vi "CheesyDrive.vi"(6 "Quickturn":bool, 10 "Wheel":dbl(slide) scale=-1.0..1.0, 11 "Throttle":dbl(slide)=-0.0 scale=-1.0..1.0) -> (2 "Right PWM":dbl=0.5949513901284444, 3 "Left PWM":dbl=0.5949513901284444)   [LabVIEW 2017]
doc: "Implements CheesyDrive. CheesyDrive means that the turn joystick controls the radius of turning instead of the rate of turning. Also implements QuickStop and QuickTurn."
panel:
  in  "Slowness":T1={"MaxSpeedSlow"=0.8, "SlowRate"=20.0, "MaxTurnSlow"=0.8, "MaxTurnRateSlow"=20.0}
  in  "PointsTurn":cluster{"X":dbl, "Y":dbl}[](array[cluster])=[{"X"=0.0, "Y"=0.0}, {"X"=0.04, "Y"=0.0}, {"X"=0.041, "Y"=0.01}, {"X"=1.0, "Y"=1.0}, {"X"=1.0, "Y"=1.0}]
  in  "PointsQuickTurn":cluster{"X":dbl, "Y":dbl}[](array[cluster])=[{"X"=0.0, "Y"=0.0}, {"X"=0.04, "Y"=0.0}, {"X"=0.7, "Y"=0.5}, {"X"=1.0, "Y"=1.0}]
  in  "PointsThrottle":cluster{"X":dbl, "Y":dbl}[](array[cluster])=[{"X"=0.0, "Y"=0.0}, {"X"=0.04, "Y"=0.0}, {"X"=0.0251, "Y"=0.15}, {"X"=1.0, "Y"=1.0}]
  in  "CarLikeTurning":bool
  in  "QSMult":dbl=0.1
  in  "WheelNonLinearity":dbl=0.65
  in  "negInertiaScalar":dbl=3.0
  in  "alpha":dbl=0.1
  out "Waveform Chart":dbl(graph)
  in  "Sensitivty":dbl=1.0
  # "Enable to enable"
  # "normal"
  # "(for quickstop decay)"
  # "Switch"
  # "Scale"
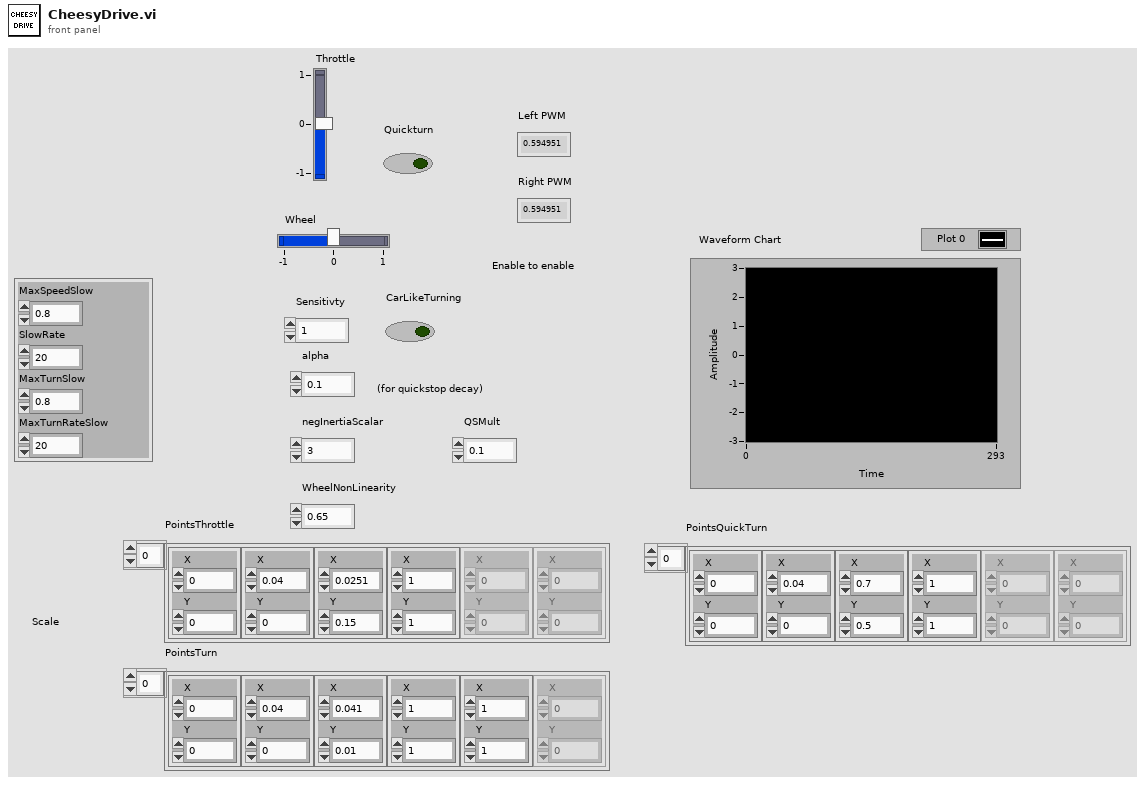
[diagram p1: front panel]
types:
  T1 = cluster{"MaxSpeedSlow":dbl, "SlowRate":dbl, "MaxTurnSlow":dbl, "MaxTurnRateSlow":dbl}
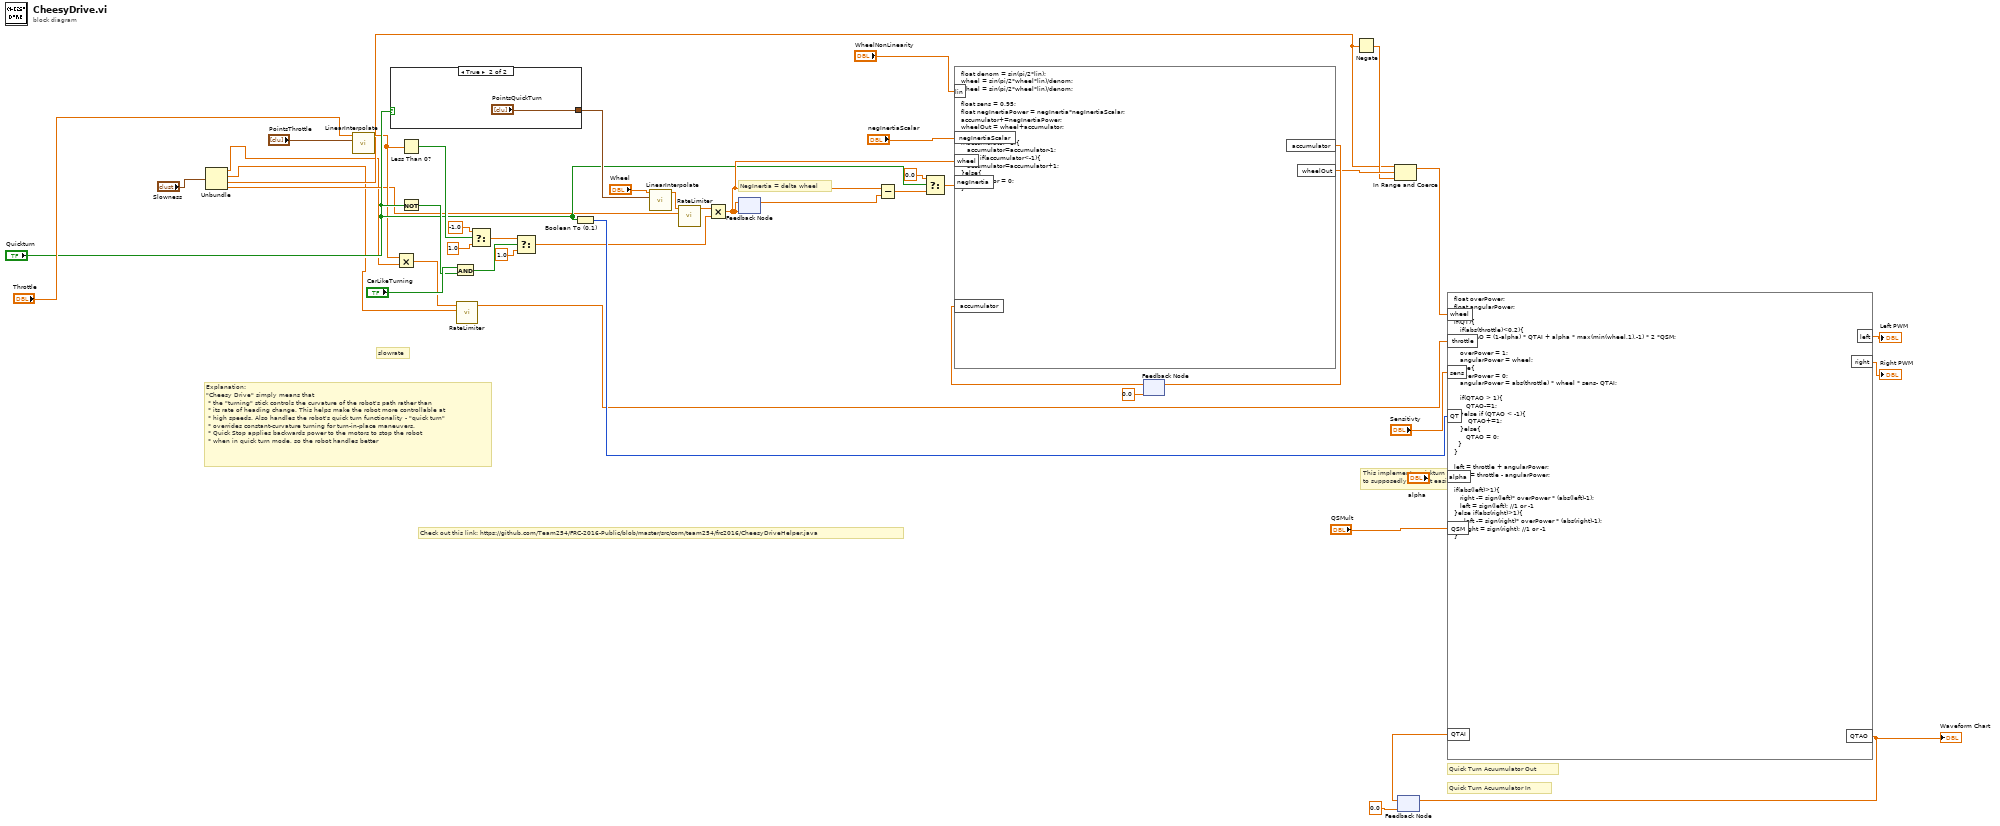
[diagram p0: block diagram]
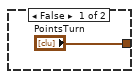
[diagram p2: hidden frame]
diagram:
  # "slowrate"
  # "This implements quickturn and also modifies wheel with a sine function\nto supposedly make it easier to drive"
  # "NegInertia = delta wheel"
  # "Explanation:\n\"Cheesy Drive\" simply means that\n * the \"turning\" stick controls the curvature of the robot's path rather than\n * its rate of heading change. This helps make the robot more controllable at\n * high speeds. Also handles the robot's quick turn functionality - \"quick turn\"\n * overrides constant-curvature turning for turn-in-place maneuvers.\n * Quick Stop applies backwards power to the motors to stop the robot\n * when in quick turn mode, so the robot handles better"
  # "Quick Turn Acuumulator Out"
  # "Quick Turn Acuumulator In"
  # "Check out this link: https://github.com/Team254/FRC-2016-Public/blob/master/src/com/team254/frc2016/CheesyDriveHelper.java"
  n1 = Unbundle("Slowness") -> ("MaxSpeedSlow"=w2:dbl, "SlowRate"=w1:dbl, "MaxTurnSlow"=w3:dbl, "MaxTurnRateSlow"=w4:dbl)
  n2 = call "LinearInterpolate.vi"("Points"="PointsThrottle", "Value"="Throttle") -> ("Output"=w7:dbl)  [unwired: 9 in]
  n3 = case shown="True" "Quickturn" {
    tunnel: ["PointsTurn" "PointsQuickTurn"] -> w20
    frame False {
    }
    frame True {
    }
  }
  n4 = Multiply(x=w7, y=w2) -> (x*y=w6:dbl)
  n5 = Less Than 0?(x=w7) -> (x < 0?=w28:bool)
  n6 = Not(x="Quickturn") -> (.not. x?=w10:bool)
  n7 = And(x="CarLikeTurning", y=w10) -> (x .and. y?=w9:bool)
  n8 = call "RateLimiter.vi"("Max dx/dt"=w1, "Input"=w6) -> ("Output"=w40:dbl)  [unwired: 9 in]
  n9 = Select(t=-1.0, s=w28, f=1.0) -> (s? t:f=w24:dbl)
  n10 = Select(t=w24, s=w9, f=1.0) -> (s? t:f=w22:dbl)
  n11 = Boolean To (0,1)(Boolean="Quickturn") -> (0, 1=w44:i16)
  n12 = call "LinearInterpolate.vi"("Points"=w20, "Value"="Wheel") -> ("Output"=w17:dbl)  [unwired: 9 in]
  n13 = call "RateLimiter.vi"("Max dx/dt"=w4, "Input"=w17) -> ("Output"=w16:dbl)  [unwired: 9 in]
  n14 = Multiply(x=w16, y=w22) -> (x*y=w25:dbl)
  n15 = feedback #1(w25) -> (w37:dbl)
  n16 = feedback-in #1(w25) -> ()
  n17 = Subtract(x=w25, y=w37) -> (x-y=w14:dbl)
  n18 = Select(t=0.0, s="Quickturn", f=w14) -> (s? t:f=w15:dbl)
  n19 = feedback #2(0.0 ("Wheel")) -> (w36:dbl)
  n20 = formula code="float denom = sin(pi/2*lin);\nwheel = sin(pi/2*wheel*lin)/denom;\nwheel = sin(pi/2*wheel*lin)/denom;\n\nfloat sens = 0.95;\nfloat negInertiaPower = negInertia*negInertiaScalar;\naccumulator+=negInertiaPower;\nwheelOut = wheel+accumulator;\n\nif(accumulator>1){\n   accumulator=accumulator-1;\n}else if(accumulator<-1){\n   accumulator=accumulator+1;\n}else{\naccumulator = 0;\n}"("wheel"=w25, "negInertia"=w15, "accumulator"=w36, "negInertiaScalar"="negInertiaScalar", "lin"="WheelNonLinearity") -> ("accumulator"=w34:dbl, "wheelOut"=w30:dbl)
  n21 = feedback-in #2(w34) -> ()
  n22 = Negate(x=w3) -> (-x=w18:dbl)
  n23 = In Range and Coerce(upper limit=w3, x=w30, lower limit=w18) -> (coerced(x)=w31:dbl)  [unwired: 1 out]
  n24 = feedback #3(0.0 ("QTAccumulatorO")) -> (w42:dbl)
  n25 = formula code="float overPower;\nfloat angularPower;\n\nif(QT){\n   if(abs(throttle)<0.2){\n      QTAO = (1-alpha) * QTAI + alpha * max(min(wheel,1),-1) * 2 *QSM;\n   }\n   overPower = 1;\n   angularPower = wheel;\n}else{\n   overPower = 0;\n   angularPower = abs(throttle) * wheel * sens- QTAI;\n\n   if(QTAO > 1){\n      QTAO-=1;\n   }else if (QTAO < -1){\n       QTAO+=1;\n   }else{\n      QTAO = 0;\n  }\n}\n\nleft = throttle + angularPower;\nright = throttle - angularPower;\n\nif(abs(left)>1){\n   right -= sign(left)* overPower * (abs(left)-1);\n   left = sign(left); //1 or -1\n}else if(abs(right)>1){\n     left -= sign(right)* overPower * (abs(right)-1);\n     right = sign(right); //1 or -1 \n}"("wheel"=w31, "throttle"=w40, "sens"="Sensitivty", "QT"=w44, "alpha"="alpha", "QTAI"=w42, "QSM"="QSMult") -> ("left"=→"Left PWM":dbl, "right"=→"Right PWM":dbl, "QTAO"=w45:dbl)
  "Waveform Chart" <- w45
  n26 = feedback-in #3(w45) -> ()
